vi "WL_Joystick GUID Lookup.vi"() -> ()   [LabVIEW 2014, in "WL_Joystick Custom Device.lvlib"]
doc: "Use this Global VI to access the GUIDs assigned to the page resources of the Custom Device."
uses:
  WL_Joystick Custom Device.lvlib
panel:
  in  "Custom Device":string="2caad80e-8be8-4562-9eb6-ca45317130ed"
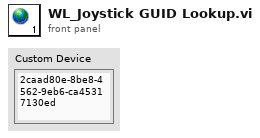
[diagram p1: front panel]
diagram:
